vi "MGI Init.vi"(10 "error":errorcluster, 11 "MGI ERD LB Row Time and Count in":refnum<class "MGI ERD LB Row Time and Count.lvclass">) -> (3 "MGI ERD LB Row Time and Count out":refnum<class "MGI ERD LB Row Time and Count.lvclass">)   [LabVIEW 2020, in "MGI ERD LB Row Time and Count.lvclass"]
doc: "Sets the Error as specified.\n\nAuthored by Shawn Walpole\nsupport@mooregoodideas.com\nwww.mooregoodideas.com\n\nCopyright (c) 2013, Moore Good Ideas, Inc.\n\nAll rights reserved.\n\nRedistribution and use in source and binary forms, with or without modification, are permitted provided that the following conditions are met:\n\n * Redistributions of source code must retain the above copyright notice, this list of conditions and the following disclaimer.\n * Redistributions in binary form must reproduce the above copyright notice, this list of conditions and the following disclaimer in the documentation and/or other materials provided with the distribution.\n * Neither the name of Moore Good Ideas, Inc. nor the names of its contributors may be used to endorse or promote products derived from this software without specific prior written permission.\n\nTHIS SOFTWARE IS PROVIDED BY THE COPYRIGHT HOLDERS AND CONTRIBUTORS \"AS IS\" AND ANY EXPRESS OR IMPLIED WARRANTIES, INCLUDING, BUT NOT LIMITED TO, THE IMPLIED WARRANTIES OF MERCHANTABILITY AND FITNESS FOR A PARTICULAR PURPOSE ARE DISCLAIMED. IN NO EVENT SHALL THE COPYRIGHT OWNER OR CONTRIBUTORS BE LIABLE FOR ANY DIRECT, INDIRECT, INCIDENTAL, SPECIAL, EXEMPLARY, OR CONSEQUENTIAL DAMAGES (INCLUDING, BUT NOT LIMITED TO, PROCUREMENT OF SUBSTITUTE GOODS OR SERVICES; LOSS OF USE, DATA, OR PROFITS; OR BUSINESS INTERRUPTION) HOWEVER CAUSED AND ON ANY THEORY OF LIABILITY, WHETHER IN CONTRACT, STRICT LIABILITY, OR TORT (INCLUDING NEGLIGENCE OR OTHERWISE) ARISING IN ANY WAY OUT OF THE USE OF THIS SOFTWARE, EVEN IF ADVISED OF THE POSSIBILITY OF SUCH DAMAGE."
uses:
  <userlib>/_MGI/Error Reporter/MGI Error Reporter Dialog/MGI ERD LB Row Time and Count/MGI ERD LB Row Time and Count.lvclass
  <userlib>/_MGI/Error Reporter/MGI Error Reporter Dialog/MGI ERD LB Row Time and Count/MGI ERD LB Row Time and Count.lvclass/MGI ERD LB Row Time and Count.ctl
  <userlib>/_MGI/Error Reporter/MGI Error Reporter Dialog/MGI ERD LB Row Base/MGI ERD LB Row Base.lvclass
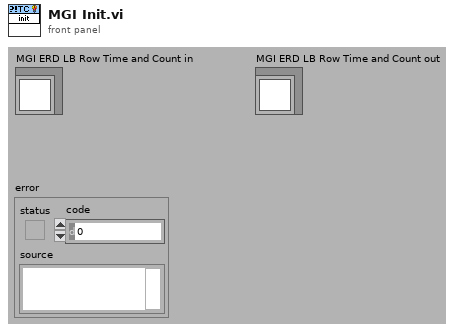
[diagram p1: front panel]
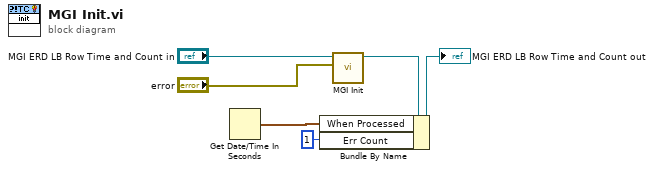
[diagram p0: block diagram]
diagram:
  n1 = Get Date/Time In Seconds() -> (seconds since 1Jan1904=w2:timestamp)
  n2 = call-parent "MGI Init.vi"("error"="error", "MGI ERD LB Row Base in"="MGI ERD LB Row Time and Count in") -> ("MGI ERD LB Row Base out"=w4:refnum<class "MGI ERD LB Row Time and Count.lvclass">)  [unwired: 9 out]
  n3 = Bundle By Name(cluster=w4, "When Processed"=w2, "Err Count"=1) -> (→"MGI ERD LB Row Time and Count out":refnum<class "MGI ERD LB Row Time and Count.lvclass">)
